vi "Global Ring Time.vi"(0 "Ring Time Plot In":waveform(dbl)(graph) caption="Ring Time Plot", 1 "Ring Time (ms) In":dbl format="%.2g", 3 "Set Data?":bool) -> (7 "Ring Time Plot Out":waveform(dbl)(graph) caption="Ring Time Plot", 8 "Ring Time (ms) Out":dbl format="%.2g")   [LabVIEW 2019]
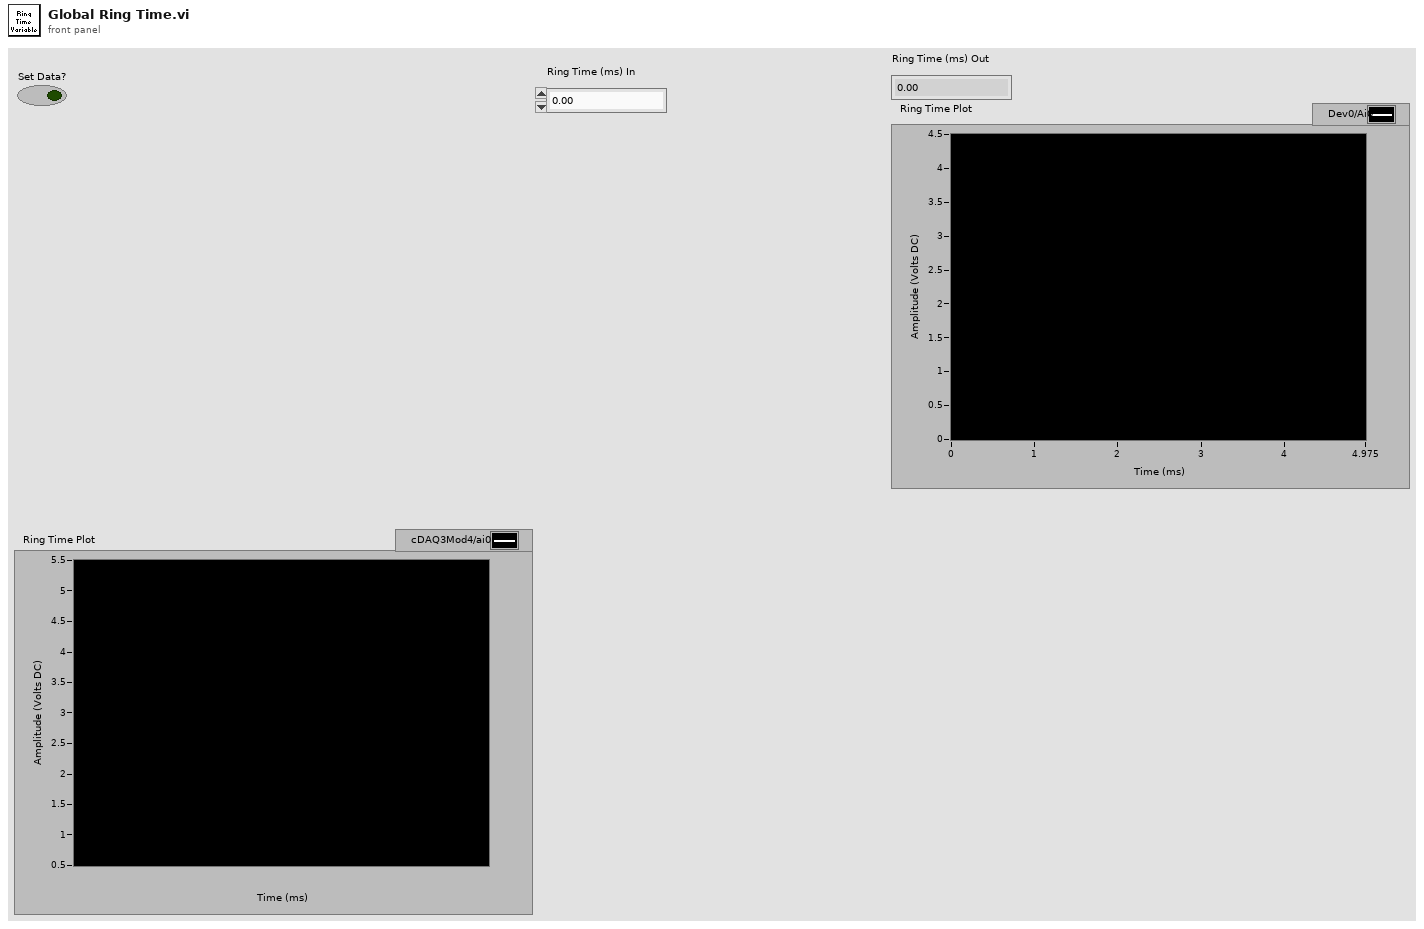
[diagram p1: front panel]
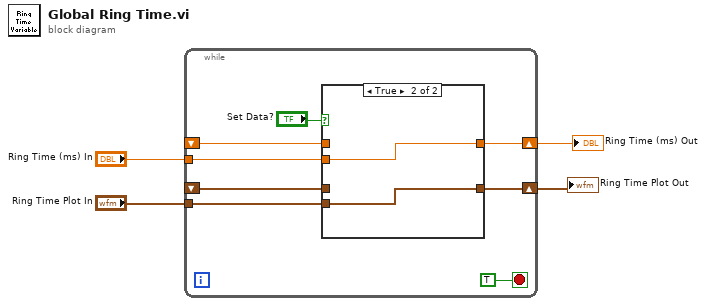
[diagram p0: block diagram]
diagram:
  n1 = while {
    shift-right: [w10] -> w3
    shift-left: _ -> [w9]
    shift-right: [w8] -> w2
    shift-left: _ -> [w7]
    tunnel: "Ring Time (ms) In" -> [w6]
    tunnel: "Ring Time Plot In" -> [w5]
    stop <- TRUE stop-if-true
    n2 = case shown="True" "Set Data?" {
      tunnel: [w14 w16] -> w10
      tunnel: w9 -> [w14 _]
      tunnel: [w13 w15] -> w8
      tunnel: w7 -> [w13 _]
      tunnel: w6 -> [_ w16]
      tunnel: w5 -> [_ w15]
      frame False {
      }
      frame True {
      }
    }
  }
  "Ring Time (ms) Out" <- w3
  "Ring Time Plot Out" <- w2
